vi "3.2.vi"() -> ()   [LabVIEW 2017]
panel:
  out "RESULT":dbl
  in  "B":dbl
  in  "A":dbl
  in  "功能选择":enum16{"相乘", "相除", "相减", "相加"}(ring)
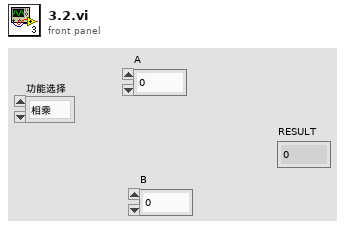
[diagram p1: front panel]
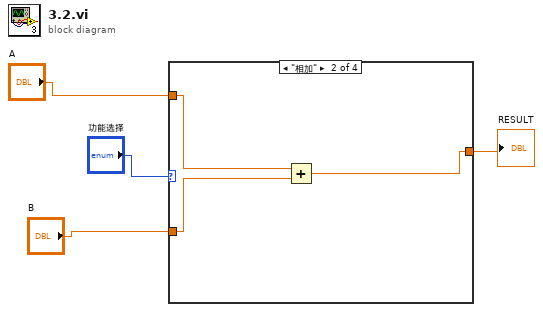
[diagram p0: block diagram]
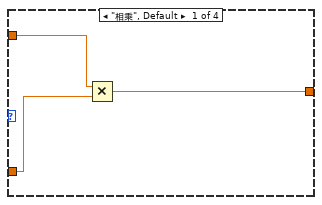
[diagram p2: hidden frame]
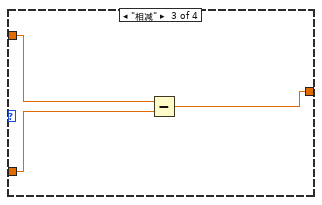
[diagram p3: hidden frame]
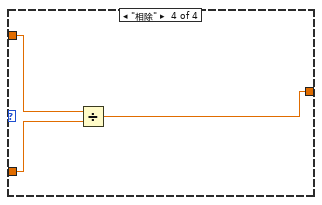
[diagram p4: hidden frame]
diagram:
  n1 = case shown="\"相加\"" "功能选择" {
    tunnel: "A" -> [w7 w10 w13 w16]
    tunnel: "B" -> [w6 w9 w12 w15]
    tunnel: [w5 w8 w11 w14] -> w1
    frame "相乘", Default {
      n2 = Multiply(x=w7, y=w6) -> (x*y=w5:dbl)
    }
    frame "相加" {
      n3 = Add(x=w10, y=w9) -> (x+y=w8:dbl)
    }
    frame "相减" {
      n4 = Subtract(x=w13, y=w12) -> (x-y=w11:dbl)
    }
    frame "相除" {
      n5 = Divide(x=w16, y=w15) -> (x/y=w14:dbl)
    }
  }
  "RESULT" <- w1
